vi "test1.vi"() -> ()   [LabVIEW 2018]
uses:
  <vilib>/imath/engines/lvmath/Plug In/_Char/NIMS_CH_character datatype.ctl
  <vilib>/imath/engines/lvmath2/RunTimeEngine/Managers/WorkSpace/UID Generator.vi
  <vilib>/imath/engines/lvmath2/RunTimeEngine/RangeToken/NIMS_Range.vi
  <instcachedir>/0/NIMS_Range_846134F467D14A349F7C6CCEF459CDB2.lvgen/NIMS_Range_846134F467D14A349F7C6CCEF459CDB2_000.vi
  <vilib>/imathl/engines/lvmath/Functions/Error Handling/Create Error.vi
  <vilib>/imath/engines/lvmath2/RunTimeEngine/RangeToken/NIMS_Range_R2 - Integer.vi
  <instcachedir>/0/NIMS_Range_R2 - Integer_E35B921DECF84AADB7325A02D418BFCC.lvgen/NIMS_Range_R2 - Integer_E35B921DECF84AADB7325A02D418BFCC_000.vi
  <vilib>/imath/engines/lvmath2/RunTimeEngine/CommandStatement/MC_CommandStatement_break.vi
  <vilib>/imath/engines/lvmath2/RunTimeEngine/BuiltInFunctions/abs/NIMS_abs(signed).vi
  <instcachedir>/0/NIMS_abs(signed)_C4FCB8E6058B49B797C7C8D53CA5F6EC.lvgen/NIMS_abs(signed)_C4FCB8E6058B49B797C7C8D53CA5F6EC_000.vi
  <vilib>/imath/engines/lvmath2/RunTimeEngine/BuiltInFunctions/bitand/NIMS_bitand(SorS,SorS).vi
  <vilib>/imath/engines/lvmath2/RunTimeEngine/IndexReplace/NIMS V(S)=S.vi
  <instcachedir>/0/NIMS V(S)=S_420DA4522869420292A92FA3CC108C4E.lvgen/NIMS V(S)=S_420DA4522869420292A92FA3CC108C4E_000.vi
  <vilib>/imath/engines/lvmath2/RunTimeEngine/BuiltInFunctions/zeros/NIMS_V=zeros(I32,I32).vi
  <vilib>/imath/engines/lvmath2/RunTimeEngine/RangeToken/NIMS_Range_R2 - Float.vi
  <instcachedir>/0/NIMS_Range_R2 - Float_6ECC2DCA6A8F4201A61F790A8BE580A7.lvgen/NIMS_Range_R2 - Float_6ECC2DCA6A8F4201A61F790A8BE580A7_000.vi
  <instcachedir>/0/NIMS V(S)=S_420DA4522869420292A92FA3CC108C4E.lvgen/NIMS V(S)=S_420DA4522869420292A92FA3CC108C4E_001.vi
  <vilib>/imath/engines/lvmath2/RunTimeSupport/NIMS_Error if Not Equal.vi
  <instcachedir>/0/NIMS_Error if Not Equal_C77461FADD9B4AE6B0EA3ED6E3A6D94D.lvgen/NIMS_Error if Not Equal_C77461FADD9B4AE6B0EA3ED6E3A6D94D_000.vi
  <vilib>/imath/engines/lvmath2/RunTimeEngine/ErrorHandling/NIMS_Create Error From Enums.vi
  <vilib>/imath/engines/lvmath2/RunTimeEngine/BuiltInFunctions/imag/NIMS_imag(Complex).vi
  <instcachedir>/0/NIMS_imag(Complex)_3180D40D00C843A49C2B33397F857BF3.lvgen/NIMS_imag(Complex)_3180D40D00C843A49C2B33397F857BF3_002.vi
  <vilib>/imath/engines/lvmath2/RunTimeEngine/RunTimeType/NIMS_RunTimeType_From StrictType (excl LVString).vi
  <instcachedir>/0/NIMS_RunTimeType_From StrictType (excl LVString)_E7E34A65C99947108168652BAD14964D.lvgen/NIMS_RunTimeType_From StrictType (excl LVString)_E7E34A65C99947108168652BAD14964D_000.vi
  <vilib>/imath/engines/lvmath2/RunTimeEngine/LocalVariableDefStatement/MC_LocalVariableDefStatement_Display.vi
  <vilib>/imath/engines/lvmath2/RunTimeEngine/BuiltInFunctions/conv/NIMS_conv(V,V).vi
  <instcachedir>/0/NIMS_conv(V,V)_D3E194F2B5174935BB2368CEB7AAC5A9.lvgen/NIMS_conv(V,V)_D3E194F2B5174935BB2368CEB7AAC5A9_000.vi
  <vilib>/imath/engines/lvmath2/RunTimeEngine/ErrorHandling/NIMS_Error From Error Code.vi
  <vilib>/imath/engines/lvmath2/RunTimeEngine/BuiltInFunctions/crosscorr/NIMS_crosscorr(GV,GV,Str).vi
  <instcachedir>/0/NIMS_crosscorr(GV,GV,Str)_A4EB815E9E924C97804DA22507CDE303.lvgen/NIMS_crosscorr(GV,GV,Str)_A4EB815E9E924C97804DA22507CDE303_001.vi
  <vilib>/imath/engines/lvmath2/RunTimeEngine/BuiltInFunctions/max/1 input/NIMS_max(RV).vi
  <instcachedir>/0/NIMS_max(RV)_237633DB1D604D5BA7001287DF3C7957.lvgen/NIMS_max(RV)_237633DB1D604D5BA7001287DF3C7957_000.vi
  <vilib>/imath/engines/lvmath2/RunTimeEngine/BuiltInFunctions/findnz/NIMS_[3o]_findnz(GRowV).vi
  <instcachedir>/0/NIMS_[3o]_findnz(GRowV)_AF5E19D8E2B0417C814DE189F19CE4A0.lvgen/NIMS_[3o]_findnz(GRowV)_AF5E19D8E2B0417C814DE189F19CE4A0_000.vi
  <vilib>/imath/engines/lvmath2/RunTimeEngine/IndexRead/NIMS V(S).vi
  <instcachedir>/0/NIMS V(S)_0488751826AF41519A22953C041130DC.lvgen/NIMS V(S)_0488751826AF41519A22953C041130DC_002.vi
  <vilib>/imath/engines/lvmath2/RunTimeEngine/BuiltInFunctions/num_to_str/NIMS_num_to_str(GRowV,I32).vi
  <instcachedir>/0/NIMS_num_to_str(GRowV,I32)_BAB3BCC9D93D469AB30EB0CE4C0C4B02.lvgen/NIMS_num_to_str(GRowV,I32)_BAB3BCC9D93D469AB30EB0CE4C0C4B02_000.vi
  <vilib>/imath/engines/lvmath/Plug In/_Char/NIMS_CH_String to Character Array.vi
  <instcachedir>/0/NIMS_RunTimeType_From StrictType (excl LVString)_E7E34A65C99947108168652BAD14964D.lvgen/NIMS_RunTimeType_From StrictType (excl LVString)_E7E34A65C99947108168652BAD14964D_001.vi
  <vilib>/imath/engines/lvmath2/RunTimeEngine/BuiltInFunctions/fft/NIMS_fft(GV).vi
  <instcachedir>/0/NIMS_fft(GV)_4C6467FC22F84E4BA42517A07EF978B0.lvgen/NIMS_fft(GV)_4C6467FC22F84E4BA42517A07EF978B0_000.vi
  <vilib>/imath/engines/lvmath2/RunTimeEngine/ArithmeticOperatorToken/NIMS_ArithmeticOperator_times.vi
  <instcachedir>/0/NIMS_ArithmeticOperator_times_D7E4A7A4AD2C4409A0CE309D2741A5B4.lvgen/NIMS_ArithmeticOperator_times_D7E4A7A4AD2C4409A0CE309D2741A5B4_003.vi
  <vilib>/imath/engines/lvmath2/RunTimeEngine/BuiltInFunctions/ifft/NIMS_ifft(CV).vi
  <vilib>/imath/engines/lvmath2/RunTimeEngine/BuiltInFunctions/hilbert/NIMS_hilbert(RV, I32).vi
  <vilib>/imath/engines/lvmath2/RunTimeEngine/Managers/SymbolTable/Clear UID.vi
  <vilib>/imath/engines/lvmath2/RunTimeEngine/NodeEndStatement/NIMS_NodeEndStatement_Output.vi
  <instcachedir>/0/NIMS_NodeEndStatement_Output_53EC0D466D134D7ABD903AC30B43404B.lvgen/NIMS_NodeEndStatement_Output_53EC0D466D134D7ABD903AC30B43404B_011.vi
  <instcachedir>/0/NIMS_NodeEndStatement_Output_53EC0D466D134D7ABD903AC30B43404B.lvgen/NIMS_NodeEndStatement_Output_53EC0D466D134D7ABD903AC30B43404B_001.vi
  <instcachedir>/0/NIMS_NodeEndStatement_Output_53EC0D466D134D7ABD903AC30B43404B.lvgen/NIMS_NodeEndStatement_Output_53EC0D466D134D7ABD903AC30B43404B_005.vi
  <vilib>/imath/engines/lvmath2/RunTimeEngine/ErrorHandling/NIMS_Finalize Error.vi
  <vilib>/imath/engines/lvmath2/RunTimeEngine/Managers/SymbolTable/NIMS_WorkSpace.lvlib
panel:
  out "T2":dbl
  out "数据变化前后对比":dbl[][](graph)
  out "D2":dbl
  out "内置函数希尔伯特变换数据":dbl[](graph)
  out "T1":dbl
  out "数据变化前后对比":dbl[][](graph)
  out "频域变化乘积所得数据":dbl[](graph)
  out "T":dbl
  out "数据变换前后对比":dbl[][](graph)
  out "D":dbl
  out "时域变化卷积所得数据":dbl[](graph)
  out "频域冲激响应":dbl[](graph)
  out "时域冲激响应":dbl[](graph)
  out "正弦信号样本":dbl[](graph)
  in  "fs":dbl=16000.0
  in  "f":dbl=1000.0
  in  "N":dbl=100.0
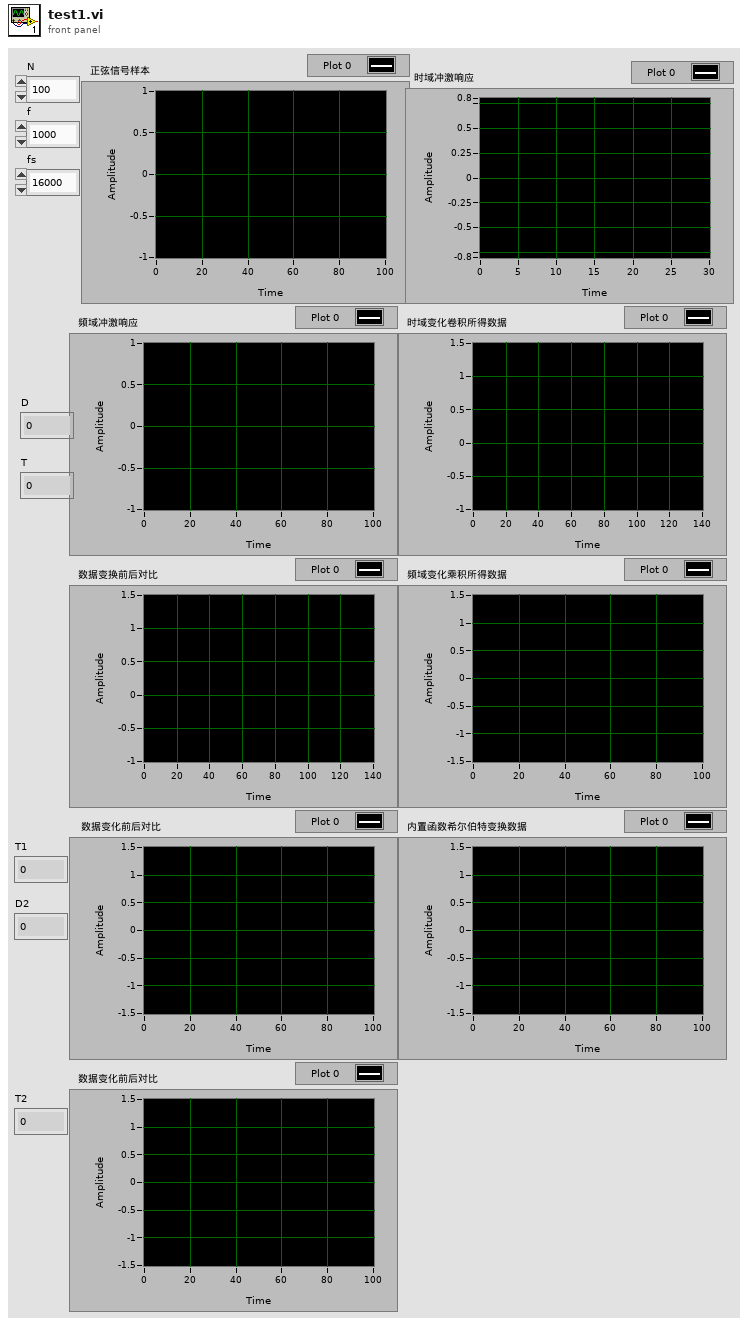
[diagram p1: front panel]
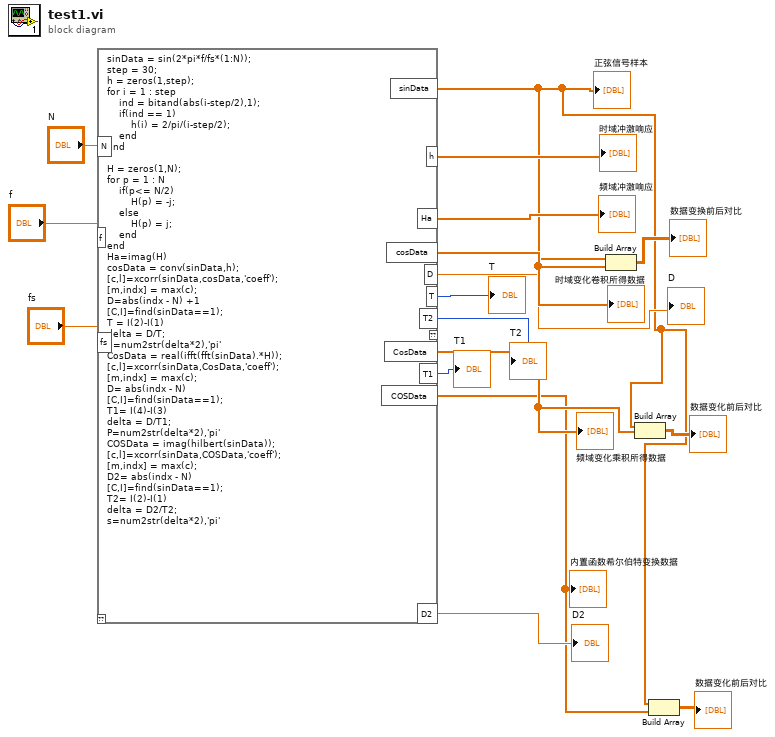
[diagram p0: block diagram]
diagram:
  n1 = mathscript code="sinData = sin(2*pi*f/fs*(1:N));\nstep = 30;\nh = zeros(1,step);\nfor i = 1 : step\n    ind = bitand(abs(i-step/2),1);\n    if(ind == 1)\n        h(i) = 2/pi/(i-step/2);\n    end\nend\n\nH = zeros(1,N);\nfor p = 1 : N\n    if(p<= N/2)\n        H(p) = -j;\n    else\n        H(p) = j;\n    end\nend\nHa=imag(H)\ncosData = conv(sinData,h);\n[c,l]=xcorr(sinData,cosData,'coeff');\n[m,indx] = max(c);\nD=abs(indx - N) +1\n[C,I]=find(sinData==1);\nT = I(2)-I(1)\ndelta = D/T;\ne=num2str(delta*2),'pi'\nCosData = real(ifft(fft(sinData).*H));\n[c,l]=xcorr(sinData,CosData,'coeff');\n[m,indx] = max(c);\nD= abs(indx - N) \n[C,I]=find(sinData==1);\nT1= I(4)-I(3)\ndelta = D/T1;\nP=num2str(delta*2),'pi'\nCOSData = imag(hilbert(sinData));\n[c,l]=xcorr(sinData,COSData,'coeff');\n[m,indx] = max(c);\nD2= abs(indx - N)\n[C,I]=find(sinData==1);\nT2= I(2)-I(1)\ndelta = D2/T2;\ns=num2str(delta*2),'pi'"("N"="N", "f"="f", "fs"="fs") -> ("sinData"=w3:dbl[], "h"=→"时域冲激响应":dbl[], "Ha"=→"频域冲激响应":dbl[], "cosData"=w12:dbl[], "T"=→"T":i32, "CosData"=w8:dbl[], "D"=→"D":dbl, "T1"=→"T1":i32, "COSData"=w4:dbl[], "D2"=→"D2":dbl, "T2"=→"T2":i32)  [unwired: 1 in, 1 out]
  "正弦信号样本" <- w3
  "时域变化卷积所得数据" <- w12
  "频域变化乘积所得数据" <- w8
  "内置函数希尔伯特变换数据" <- w4
  n2 = Build Array(w3, w12) -> (→"数据变换前后对比":dbl[][])
  n3 = Build Array(w3, w8) -> (→"数据变化前后对比":dbl[][])
  n4 = Build Array(w3, w4) -> (→"数据变化前后对比":dbl[][])
